vi "ReadTime.vi"() -> (0 "element":dbl)   [LabVIEW 2013]
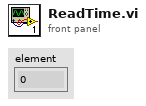
[diagram p1: front panel]
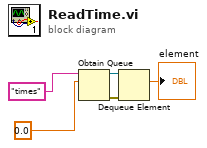
[diagram p0: block diagram]
diagram:
  n1 = Obtain Queue(name (unnamed)="times", element data type=0.0) -> (queue out=w4:refnum<queue>, error out=w3:errorcluster)  [unwired: 3 in, 1 out]
  n2 = Dequeue Element(queue=w4, error in (no error)=w3) -> (element=→"element":dbl)  [unwired: 1 in, 3 out]
